vi "FPGA_main_v3.vi"() -> ()   [LabVIEW 2018]
doc: "FPGA main VI for AI input and output.\n\nSamples at 100 kHz and downsamples to 1 kHz."
uses:
  <vilib>/rvi/Emulation/niFpgaGetClockAttributes.vi
  <vilib>/rvi/Emulation/niFpgaSctlEmulationGetInTimedLoop.vi
  <vilib>/rvi/Emulation/niFpgaEmulationReportErrorSimple.vi
  <vilib>/rvi/eio/common/nirviEmuTemplateMethod_errors.vi
  <vilib>/rvi/Emulation/niFpgaEmulationIsFPGAContextNoSignature.vi
  <vilib>/rvi/errors/niFpgaSetErrorForExecOnDevCompSimple.vi
  <vilib>/rvi/eio/common/nirviEmuReportErrorAndStop.vi
  <vilib>/rvi/DataTransferAndStorage/Container/Common/niFpgaContainerGetUniqueNameForEmu.vi
  <vilib>/rvi/FIFO/Fifo_Resource/nirvififoEmulationSetSize.vi
  <vilib>/rvi/FIFO/Fifo_Resource/nirviFifoEmulationQueueMgr.vi
  <instcachedir>/0/nirviFifoEmulationQueueMgr_E5CAEC123FF24DC58D834DCA3CDAA9B5.lvgen/nirviFifoEmulationQueueMgr_E5CAEC123FF24DC58D834DCA3CDAA9B5_003.vi
  <vilib>/rvi/FIFO/Fifo_Resource/nirvififoEmulationDetermineInputValidOut.vi
  <vilib>/rvi/FIFO/Fifo_Resource/nirvififoEmulationCreateLock.vi
  <vilib>/rvi/Emulation/niFpgaProcessEmulError.vi
  <vilib>/rvi/FIFO/Fifo_Resource/nirvififoEmulationObtainLock.vi
  <vilib>/rvi/FIFO/Fifo_Resource/nirvififoEmulationReleaseLock.vi
  <vilib>/rvi/occurrence/nirviWaitOnOccurrenceBase.vi
  <vilib>/rvi/errors/nirviReportUnexpectedCaseInternalError.vi
  <vilib>/rvi/errors/nirviReportUnexpectedCaseInternalError (U32).vi
  <vilib>/rvi/Emulation/niFpgaCriticalErrorInLSC.vi
  <vilib>/Utility/error.llb/Clear Errors.vi
  <vilib>/eio/EIONode/EIONode.xnode
  <vilib>/rvi/DataTransferAndStorage/Container/XNode/niFpgaContainer.xnode
  <vilib>/rvi/FIFO/Fifo_Resource/nirvififoEmulationWrite.vi
  <vilib>/rvi/FIFO/Fifo_Resource/nirvififoEmulationRead.vi
  Components/FPGA functions/FPGA functions.lvlib
panel:
  in  "I/O sample time (us)":u8=3
  out "LPF loop rate (us)":u8
  out "ConnectorC/AI0":fxp<+/-,22,5> format="%#_7g"
  out "Signal I/O loop rate (us)":u8
  in  "ConnectorC/AO0":i16
  # "Inputs"
  # "Sampling time"
  # "Filtered AI"
  # "For each additional bit of resolution, the signal must be oversampled by a factor of four:\nf_os = 4^w f_s \nwhere w is the number of additional bits of resolution desired, f_s is the original sampling frequency requirement, and f_os is the oversampling frequency\n\nhttp://www.cypress.com/file/236481/download"
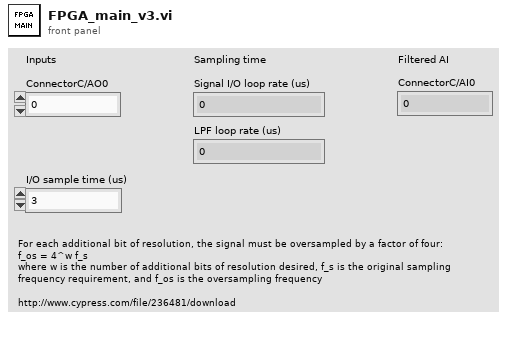
[diagram p1: front panel]
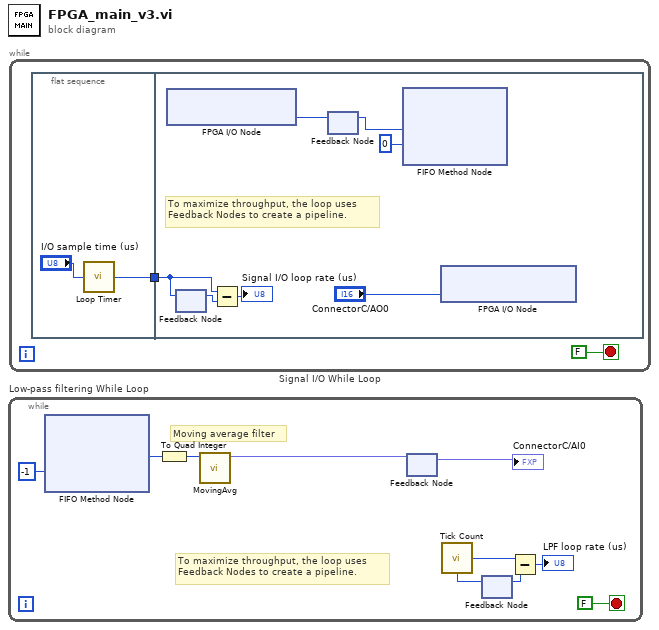
[diagram p0: block diagram]
diagram:
  n1 = while "Low-pass filtering While Loop" {
    stop <- FALSE stop-if-true
    # "Moving average filter"
    # "To maximize throughput, the loop uses \nFeedback Nodes to create a pipeline."
    n2 = xnode ("FIFO Method Node")("Timeout"=-1) -> ("Element"=w3:i16)  [unwired: 1 in, 2 out]
    n3 = To Quad Integer(1:w3) -> (0:w4:i64)
    n4 = call "MovingAvg.vi"("Raw Voltage Input [Int.]"=w4) -> ("Analog Volt Out [FXP.]"=w2:fxp<+/-,22,5>)  [unwired: 10 in]
    n5 = feedback #1() -> (→"ConnectorC/AI0":fxp<+/-,22,5>)  [unwired: 1 in]
    n6 = feedback-in #1(w2) -> ()
    n7 = call "Tick Count"() -> ("Tick Count(uSec)"=w7:u8)
    n8 = feedback-in #2(w7) -> ()
    n9 = feedback #2() -> (w6:u8)  [unwired: 1 in]
    n10 = Subtract(x=w7, y=w6) -> (x-y=→"LPF loop rate (us)":u8)
  }
  n11 = while "Signal I/O While Loop" {
    stop <- FALSE stop-if-true
    n12 = flat-sequence {
      tunnel: [w13] -> w10
      tunnel: w10 -> [w19]
      frame #0 {
        n13 = call "Loop Timer"("Count(uSec)"="I/O sample time (us)") -> ("Tick Count(uSec)"=w13:u8)
      }
      frame #1 {
        # "To maximize throughput, the loop uses \nFeedback Nodes to create a pipeline."
        n14 = xnode "FPGA I/O Node"() -> ("ConnectorC/AI0"=w17:i16)  [unwired: 1 in, 1 out]
        n15 = feedback #3() -> (w20:u8)  [unwired: 1 in]
        n16 = feedback-in #3(w19) -> ()
        n17 = Subtract(x=w19, y=w20) -> (x-y=→"Signal I/O loop rate (us)":u8)
        n18 = feedback-in #4(w17) -> ()
        n19 = feedback #4() -> (w15:i16)  [unwired: 1 in]
        n20 = xnode ("FIFO Method Node")("Element"=w15, "Timeout"=0) -> ()  [unwired: 1 in, 2 out]
        n21 = xnode "FPGA I/O Node"("ConnectorC/AO0"="ConnectorC/AO0") -> ()  [unwired: 1 in, 1 out]
      }
    }
  }
